vi "Set Error (Scope).vi"(8 "error in (no error)":errorcluster, 9 "error list <scope>":variant, 10 "scope":T1, 11 "error list <top> in":variant) -> (0 "error out":errorcluster, 3 "error list <top> out":variant)   [LabVIEW 2017]
uses:
  Scope.ctl
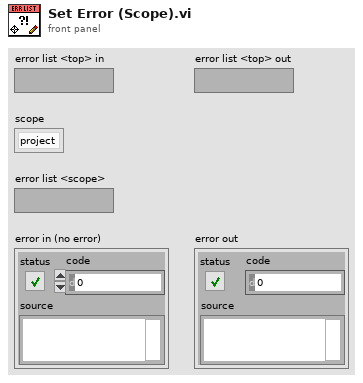
[diagram p1: front panel]
types:
  T1 = typedef "Scope.ctl" = enum16{"project", "global"}
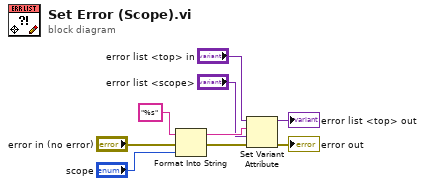
[diagram p0: block diagram]
diagram:
  n1 = Format Into String(format string="%s", error in="error in (no error)", "scope") -> (resulting string=w7:string, error out=w8:errorcluster)  [unwired: 1 in]
  n2 = Set Variant Attribute(Variant="error list <top> in", name=w7, value="error list <scope>", error in=w8) -> (Variant out=→"error list <top> out":variant, error out=→"error out":errorcluster)  [unwired: 1 out]
